vi "SpecCurveData.vi"(4 "spectal data":dbl[](array[numeric]) format="%.2f", 6 "Fit band":T3 {"center freq" format="%.2f"; "stop freq" format="%.2f"; "start freq" format="%.2f"}, 7 "Fit params":T4 {"pts in fit" format="%.2f"; "midband fit" format="%.2f"; "intercept (b)" format="%.2f"; "slope (m)" format="%.2f"}, 8 "Array Subset":T1, 9 "delay":sgl format="%.2f", 10 "sample rate MHz":u16, 11 "RF Info":T2) -> (3 "Spectra data":string)   [LabVIEW 2022 SP3]
panel:
  # "Convert data into a string with"
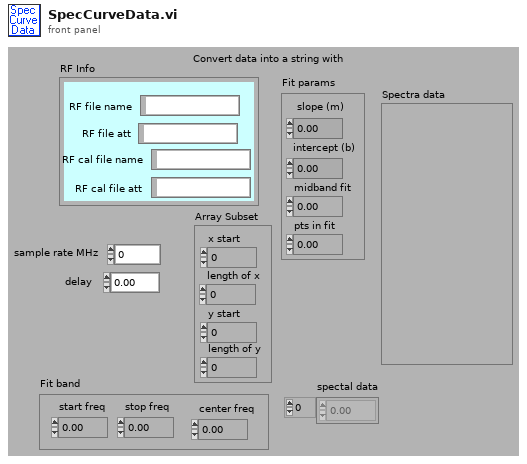
[diagram p1: front panel]
types:
  T1 = cluster{"x start":i32, "length of x":i32, "y start":i32, "length of y":i32}
  T2 = cluster{"RF file name":string, "RF file att":string, "RF cal file name":string, "RF cal file att":string}
  T3 = cluster{"start freq":dbl, "stop freq":dbl, "center freq":dbl}
  T4 = cluster{"slope (m)":dbl, "intercept (b)":dbl, "midband fit":dbl, "pts in fit":dbl}
  T5 = cluster{"x start":string, "length of x":string, "y start":string, "length of y":string}
  T6 = cluster{"slope (m)":string, "intercept (b)":string, "midband fit":string, "pts in fit":string}
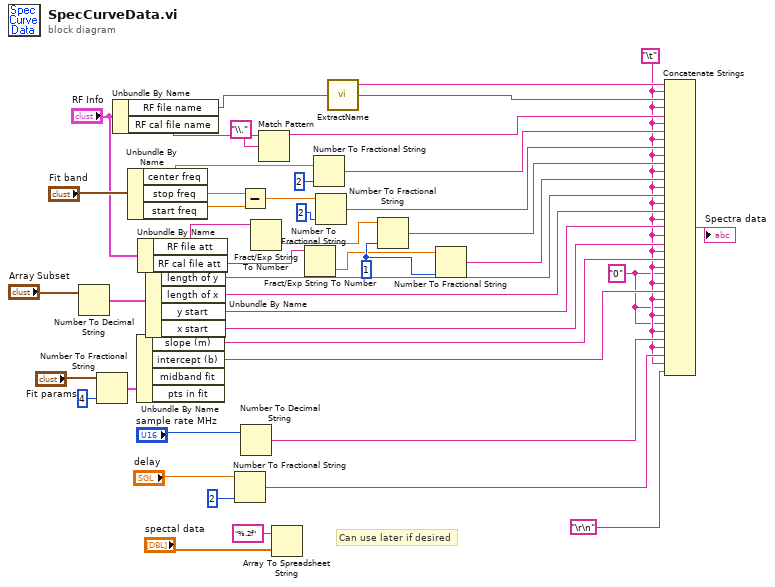
[diagram p0: block diagram]
diagram:
  w1 = "0"
  w7 = 1
  w2 = "\t"
  # "Can use later if desired"
  n1 = Number To Decimal String(number="Array Subset") -> (decimal integer string=w33:T5)  [unwired: 1 out]
  n2 = Number To Fractional String(number="Fit params", precision (6)=i16 4) -> (F-format string=w28:T6)  [unwired: 2 out]
  n3 = Unbundle By Name("RF Info") -> ("RF file name"=w16:string, "RF cal file name"=w36:string)
  n4 = Unbundle By Name("Fit band") -> ("center freq"=w41:dbl, "stop freq"=w43:dbl, "start freq"=w42:dbl)
  n5 = Unbundle By Name(w28) -> ("slope (m)"=w23:string, "intercept (b)"=w26:string)  [unwired: 2 out]
  n6 = Unbundle By Name("RF Info") -> ("RF file att"=w11:string, "RF cal file att"=w10:string)
  n7 = Unbundle By Name(w33) -> ("length of y"=w32:string, "length of x"=w31:string, "y start"=w30:string, "x start"=w29:string)
  n8 = Number To Fractional String(number="delay", precision (6)=2) -> (F-format string=w12:string)  [unwired: 2 out]
  n9 = Subtract(x=w43, y=w42) -> (x-y=w40:dbl)
  n10 = Number To Decimal String(number="sample rate MHz") -> (decimal integer string=w13:string)  [unwired: 1 out]
  n11 = Fract/Exp String To Number(string=w11) -> (number=w6:dbl)  [unwired: 4 out]
  n12 = Match Pattern(string=w36, regular expression="\\." ("string")) -> (before substring=w39:string)  [unwired: 4 out]
  n13 = Array To Spreadsheet String(array="spectal data", 3:"%.2f" ("format string")) -> ()  [unwired: 2 out]
  n14 = Fract/Exp String To Number(string=w10) -> (number=w5:dbl)  [unwired: 4 out]
  n15 = Number To Fractional String(number=w41, precision (6)=i16 2) -> (F-format string=w38:string)  [unwired: 2 out]
  n16 = Number To Fractional String(number=w40, precision (6)=i16 2) -> (F-format string=w37:string)  [unwired: 2 out]
  n17 = call "ExtractName.vi"("Full File Name"=w16) -> ("Root File Name"=w14:string, "File Number"=w15:string)  [unwired: 1 out]
  n18 = Number To Fractional String(number=w6, precision (6)=w7) -> (F-format string=w9:string)  [unwired: 2 out]
  n19 = Number To Fractional String(number=w5, precision (6)=w7) -> (F-format string=w8:string)  [unwired: 2 out]
  n20 = Concatenate Strings(w14, w2, w15, w2, w39, w2, w38, w2, w37, w2, w9, w2, w8, w2, w32, w2, w31, w2, w30, w2, w29, w2, w23, w2, w1, w2, w26, w2, w1, w2, w1, w2, w13, w2, w12, w2, "\r\n") -> (→"Spectra data":string)
